vi "editscenario format Post to Scenario.vi"(6 "User Information":T2, 8 "error in (no error)":errorcluster, 9 "Scenario (none)":T3, 10 "Save POST":T6, 11 "Connection Ref":T1) -> (0 "error out":errorcluster, 1 "new Scenario":T3, 2 "Overwrite ixScenario":i32, 3 "dup Connection Ref":T1)   [LabVIEW 2011]
uses:
  Addons/internet/utils/keyedarr.llb/Keyed Array.ctl
  server/database/Scenarios/Scenario Record.ctl
  server/database/Scenarios/Conditions/Condition Record.ctl
  server/database/Scenarios/Conditions/Condition Operators.ctl
  server/database/Users/User Record.ctl
  SI.LIB/ODBC/SQL Controls/Connection Refnum.ctl
  Addons/internet/utils/strutil.llb/Case Matching.ctl
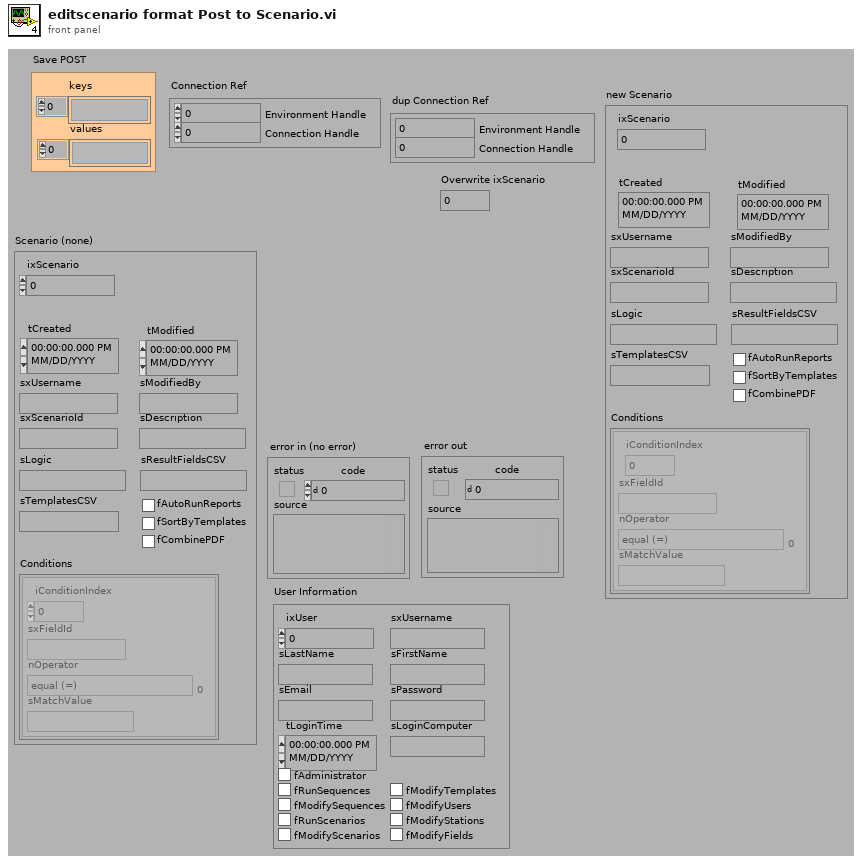
[diagram p1: front panel]
types:
  T1 = typedef "Connection Refnum.ctl" = cluster{"Environment Handle":i32, "Connection Handle":i32}
  T2 = typedef "User Record.ctl" = cluster{"ixUser":i32, "sxUsername":string, "sLastName":string, "sFirstName":string, "sEmail":string, "sPassword":string, "tLoginTime":timestamp, "sLoginComputer":string, "fAdministrator":bool, "fRunSequences":bool, "fModifySequences":bool, "fRunScenarios":bool, "fModifyScenarios":bool, "fModifyTemplates":bool, "fModifyUsers":bool, "fModifyStations":bool, "fModifyFields":bool}
  T3 = typedef "Scenario Record.ctl" = cluster{"ixScenario":i32, "tCreated":timestamp, "tModified":timestamp, "sxUsername":string, "sModifiedBy":string, "sxScenarioId":string, "sDescription":string, "sLogic":string, "sResultFieldsCSV":string, "sTemplatesCSV":string, "fAutoRunReports":bool, "fSortByTemplates":bool, "fCombinePDF":bool, "Conditions":T4[]}
  T4 = typedef "Condition Record.ctl" = cluster{"iConditionIndex":i32, "sxFieldId":string, "nOperator":T5, "sMatchValue":string}
  T5 = typedef "Condition Operators.ctl" = enum16{"equal (=)", "not equal (\\u2260)", "less than (<)", "less than or equal (\\u2264)", "greater than (>)", "greater than or equal (\\u2265)", "contains", "does not contain"}
  T6 = typedef "Keyed Array.ctl" = cluster{"keys":string[], "values":string[]}
  T7 = typedef "Case Matching.ctl" = enum16{"a != A", "a == A", "system"}
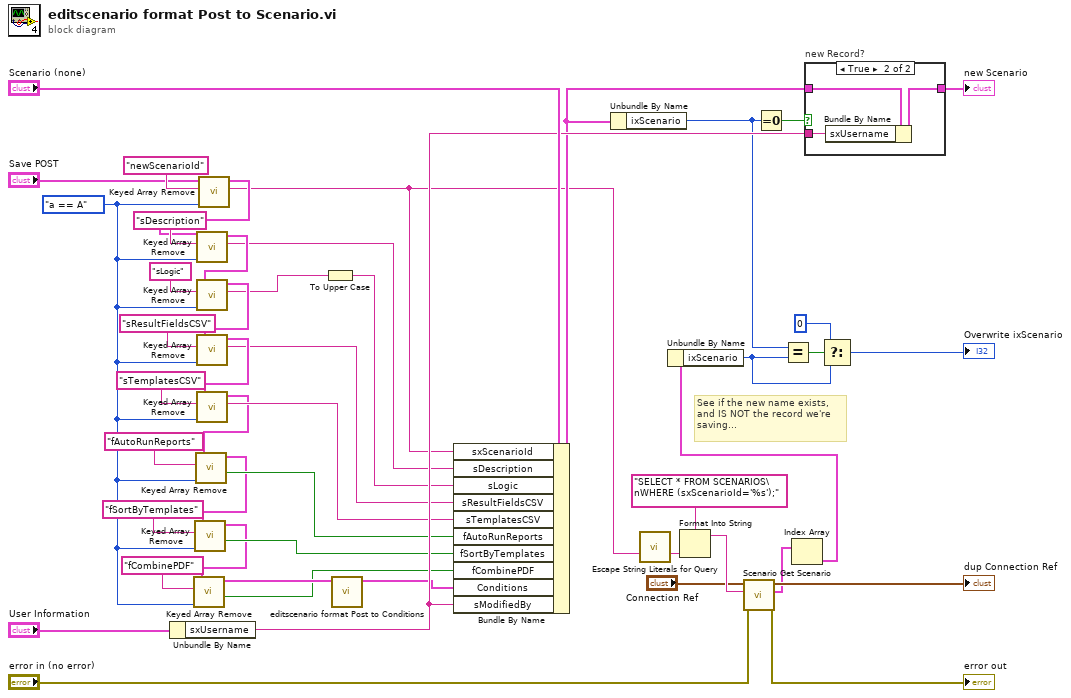
[diagram p0: block diagram]
diagram:
  w17 = Case_Matching."a == A" ("case matching (sensitive)")
  # "See if the new name exists,\nand IS NOT the record we're\nsaving..."
  n1 = Unbundle By Name("User Information") -> ("sxUsername"=w40:string)
  n2 = call "Keyed Array Remove.vi"("case matching (sensitive)"=w17, "key"="newScenarioId", "array in"="Save POST") -> ("value"=w13:string, "array out"=w18:T6)  [unwired: 3 out]
  n3 = call "Keyed Array Remove.vi"("case matching (sensitive)"=w17, "key"="sDescription", "array in"=w18) -> ("value"=w34:string, "array out"=w45:T6)  [unwired: 3 out]
  n4 = call "Keyed Array Remove.vi"("case matching (sensitive)"=w17, "key"="sLogic", "array in"=w45) -> ("value"=w33:string, "array out"=w42:T6)  [unwired: 3 out]
  n5 = call "Keyed Array Remove.vi"("case matching (sensitive)"=w17, "key"="sResultFieldsCSV", "array in"=w42) -> ("value"=w32:string, "array out"=w35:T6)  [unwired: 3 out]
  n6 = call "Keyed Array Remove.vi"("case matching (sensitive)"=w17, "key"="sTemplatesCSV", "array in"=w35) -> ("value"=w31:string, "array out"=w22:T6)  [unwired: 3 out]
  n7 = call "Keyed Array Remove.vi"("case matching (sensitive)"=w17, "key"="fAutoRunReports", "array in"=w22) -> ("valid key"=w23:bool, "array out"=w21:T6)  [unwired: 3 out]
  n8 = call "Keyed Array Remove.vi"("case matching (sensitive)"=w17, "key"="fSortByTemplates", "array in"=w21) -> ("valid key"=w29:bool, "array out"=w27:T6)  [unwired: 3 out]
  n9 = call "Keyed Array Remove.vi"("case matching (sensitive)"=w17, "key"="fCombinePDF", "array in"=w27) -> ("valid key"=w25:bool, "array out"=w26:T6)  [unwired: 3 out]
  n10 = To Upper Case(1:w33) -> (0:w37:string)
  n11 = call "editscenario format Post to Conditions.vi"("Save POST"=w26) -> ("Conditions"=w38:T4[])  [unwired: 10 out]
  n12 = Bundle By Name(cluster="Scenario (none)", "sxScenarioId"=w13, "sDescription"=w34, "sLogic"=w37, "sResultFieldsCSV"=w32, "sTemplatesCSV"=w31, "fAutoRunReports"=w23, "fSortByTemplates"=w29, "fCombinePDF"=w25, "Conditions"=w38, "sModifiedBy"=w40) -> (w16:T3)
  n13 = Unbundle By Name(w16) -> ("ixScenario"=w5:i32)
  n14 = call "Escape String Literals for Query.vi"("String"=w13) -> ("escaped String"=w15:string)  [unwired: 1 in, 13 out]
  n15 = Format Into String(format string="SELECT * FROM SCENARIOS\nWHERE (sxScenarioId='%s');", w15) -> (resulting string=w14:string)  [unwired: 2 in, 1 out]
  n16 = call "Scenario Get Scenario.vi"("error in (no error)"="error in (no error)", "Query"=w14, "Connection Refnum"="Connection Ref") -> ("error out"=→"error out":errorcluster, "Scenarios"=w7:T3[], "Connection Refnum"=→"dup Connection Ref":T1)  [unwired: 6 out]
  n17 = Equal To 0?(x=w5) -> (x = 0?=w41:bool)
  n18 = Index Array(array=w7) -> (element=w6:T3)  [unwired: 1 in]
  n19 = Unbundle By Name(w6) -> ("ixScenario"=w2:i32)
  n20 = Equal?(x=w5, y=w2) -> (x = y?=w4:bool)
  n21 = case "new Record?" shown="True" w41 {
    tunnel: w16 -> [w49 w52]
    tunnel: w40 -> [_ w51]
    tunnel: [w49 w50] -> w39
    frame False {
    }
    frame True {
      n22 = Bundle By Name(cluster=w52, "sxUsername"=w51) -> (w50:T3)
    }
  }
  "new Scenario" <- w39
  n23 = Select(t=0, s=w4, f=w2) -> (s? t:f=→"Overwrite ixScenario":i32)
